vi "teraterm_console.vi"(7 "teraterm ini template":string, 8 "error in (no error)":errorcluster, 9 "Options":T1, 10 "Com port num (COMxxx)":string, 11 "Console number (1)":u32=1 min=1 step=1) -> (0 "error out":errorcluster)   [LabVIEW 2013]
uses:
  Test Support VI/Tera term Serial options.ctl
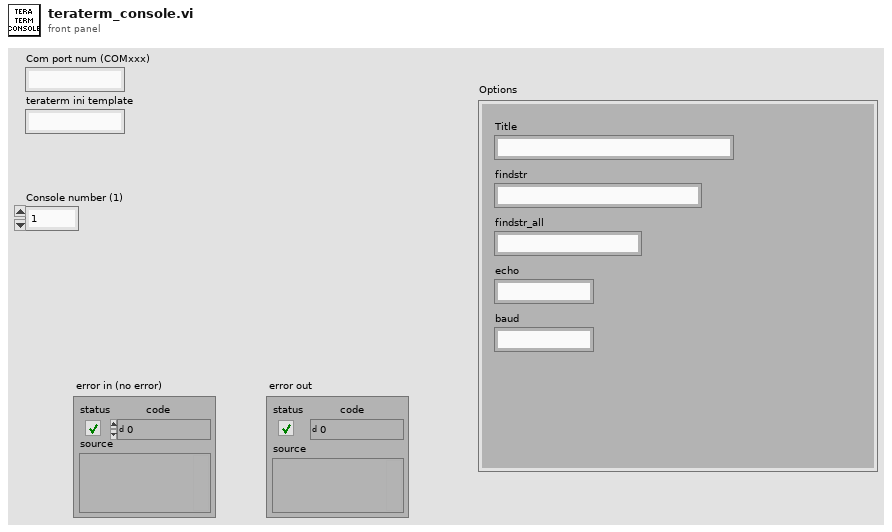
[diagram p1: front panel]
types:
  T1 = typedef "Tera term Serial options.ctl" = cluster{"Title":string, "findstr":string, "findstr_all":string, "echo":string, "baud":string}
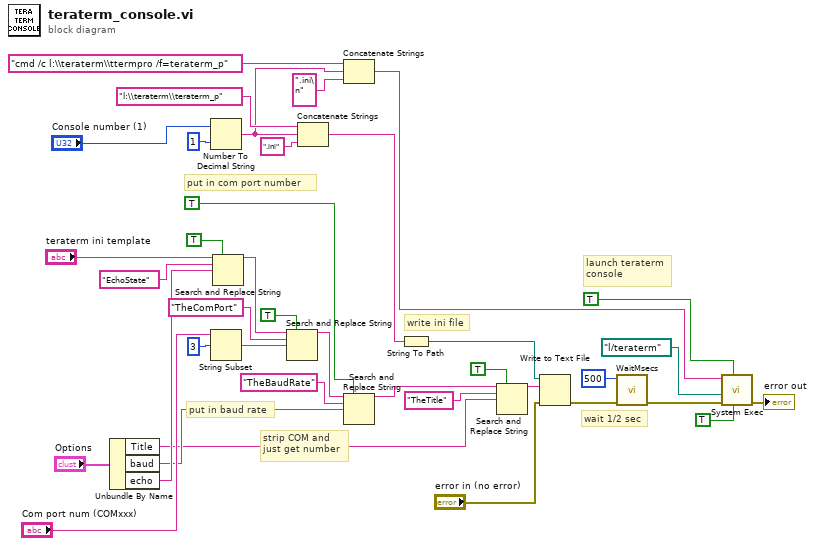
[diagram p0: block diagram]
diagram:
  # "write ini file"
  # "put in com port number"
  # "put in baud rate"
  # "launch teraterm\nconsole"
  # "wait 1/2 sec"
  # "strip COM and\njust get number"
  n1 = Unbundle By Name("Options") -> ("Title"=w2:string, "baud"=w6:string, "echo"=w7:string)
  n2 = Number To Decimal String(number="Console number (1)", width (-)=i16 1) -> (decimal integer string=w12:string)
  n3 = String Subset(string="Com port num (COMxxx)", offset (0)=3) -> (substring=w18:string)  [unwired: 1 in]
  n4 = Search and Replace String(replace all?=TRUE ("replace all? (F)"), input string="teraterm ini template", search string="EchoState", replace string=w7) -> (result string=w30:string)  [unwired: 4 in, 3 out]
  n5 = Search and Replace String(replace all?=TRUE ("replace all? (F)"), input string=w30, search string="TheComPort", replace string=w18) -> (result string=w25:string)  [unwired: 4 in, 3 out]
  n6 = Concatenate Strings("l:\\teraterm\\teraterm_p", w12, ".ini") -> (w10:string)
  n7 = Concatenate Strings("cmd /c l:\\teraterm\\ttermpro /f=teraterm_p", w12, ".ini\n") -> (w15:string)
  n8 = Search and Replace String(replace all?=TRUE ("replace all? (F)"), input string=w25, search string="TheBaudRate", replace string=w6) -> (result string=w3:string)  [unwired: 4 in, 3 out]
  n9 = String To Path(string=w10) -> (path=w9:path)
  n10 = Search and Replace String(replace all?=TRUE ("replace all? (F)"), input string=w3, search string="TheTitle", replace string=w2) -> (result string=w1:string)  [unwired: 4 in, 3 out]
  n11 = Write to Text File(file (use dialog)=w9, text=w1, error in="error in (no error)") -> (error out=w23:errorcluster)  [unwired: 1 in, 2 out]
  n12 = call "WaitMsecs.vi"("error in (no error)"=w23, "Wait Msecs"=u32 500) -> ("error out"=w21:errorcluster)  [unwired: 9 in]
  n13 = call <vilib>:"System Exec.vi"("run minimized? (F)"=TRUE, "wait until completion? (T)"=TRUE, "error in (no error)"=w21, "working directory"=path "l:/teraterm", "command line"=w15) -> ("error out"=→"error out":errorcluster)  [unwired: 3 in, 3 out]
